vi "Init.vi"(7 "I2C #":T1=-1, 8 "error in (no error)":errorcluster, 10 "Session In":refnum<class "Session.lvclass">) -> (0 "error out":errorcluster, 3 "DFRobot_Gravity_GNSS Out":refnum<class "DFRobot_Gravity_GNSS.lvclass">)   [LabVIEW 2020, in "CTI-Peripheral.lvlib" / "DFRobot_Gravity_GNSS.lvclass"]
uses:
  DFRobot_Gravity_GNSS.lvclass
  CTI/Session/Session.lvclass
  CTI/I2C Number.ctl
  CTI/I2C Address.ctl
  CTI/I2C Connection/I2C Connection.lvclass/I2C Connection.ctl
  DFRobot_Gravity_GNSS.lvclass/DFRobot_Gravity_GNSS.ctl
  CTI/I2C Connection/I2C Connection.lvclass
  CTI/CTI.lvlib
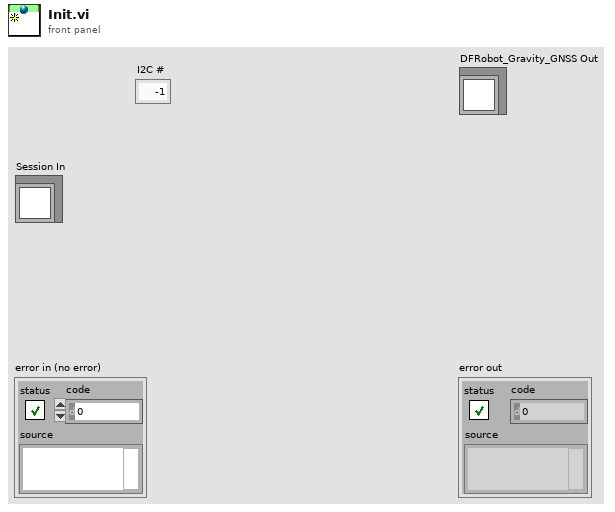
[diagram p1: front panel]
types:
  T1 = typedef "CTI.lvlib/I2C Number.ctl" = i8
  T2 = typedef "CTI.lvlib/I2C Address.ctl" = u8
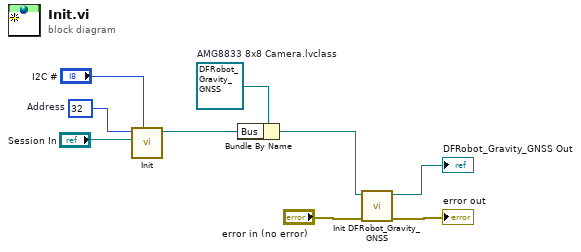
[diagram p0: block diagram]
diagram:
  w5 = refnum<class "DFRobot_Gravity_GNSS.lvclass"> refnum  # AMG8833 8x8 Camera.lvclass
  w6 = T2 32  # Address
  n1 = call "Init.vi"("I2C #"="I2C #", "Session"="Session In", "Address"=w6) -> ("I2C Connection"=w9:refnum<class "I2C Connection.lvclass">)  [unwired: 7 in, 1 out]
  n2 = Bundle By Name(cluster=w5, "Bus"=w9) -> (w4:refnum<class "DFRobot_Gravity_GNSS.lvclass">)
  n3 = call "Init DFRobot_Gravity_GNSS.vi"("error in (no error)"="error in (no error)", "DFRobot_Gravity_GNSS in"=w4) -> ("error out"=→"error out":errorcluster, "DFRobot_Gravity_GNSS out"=→"DFRobot_Gravity_GNSS Out":refnum<class "DFRobot_Gravity_GNSS.lvclass">)  [unwired: 8 in]
